vi "read_data.vi"(8 "error in (no error)":errorcluster, 11 "FeatureAgglomeration in":refnum<class "FeatureAgglomeration.lvclass">) -> (0 "error out":errorcluster, 2 "data":T1, 3 "FeatureAgglomeration out":refnum<class "FeatureAgglomeration.lvclass">)   [LabVIEW 2020, in "FeatureAgglomeration.lvclass"]
uses:
  FeatureAgglomeration.lvclass
  Controls/feature_agglomeration_data.ctl
  FeatureAgglomeration.lvclass/FeatureAgglomeration.ctl
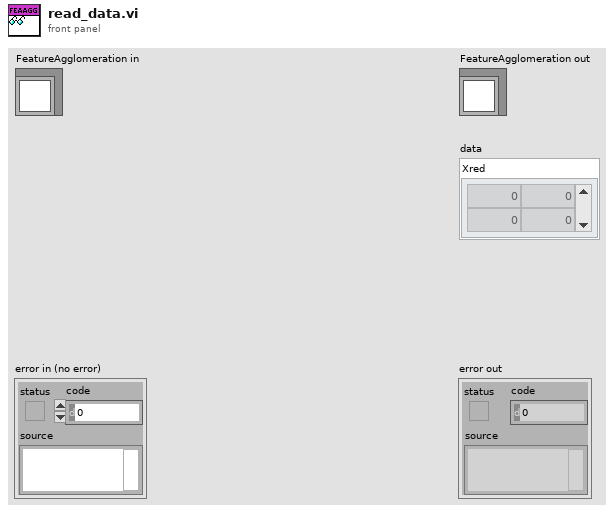
[diagram p1: front panel]
types:
  T1 = typedef "feature_agglomeration_data.ctl" = cluster{"Xred":dbl[][]}
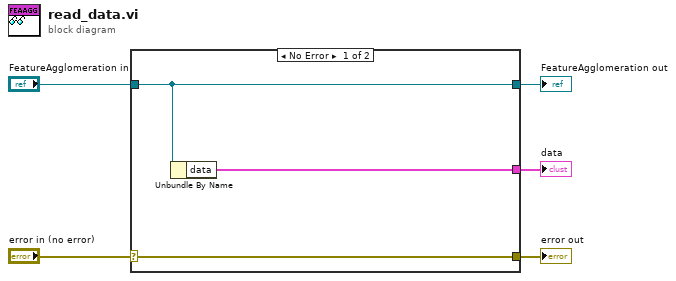
[diagram p0: block diagram]
diagram:
  n1 = case shown="No Error" "error in (no error)" {
    selector: "error in (no error)" -> [w8 w9]
    tunnel: [w8 w9] -> w4
    tunnel: [w7 w10] -> w2
    tunnel: "FeatureAgglomeration in" -> [w7 w10]
    tunnel: [w6 _] -> w1
    frame No Error {
      n2 = Unbundle By Name(w7) -> ("data"=w6:T1)
    }
    frame Error {
    }
  }
  "error out" <- w4
  "FeatureAgglomeration out" <- w2
  "data" <- w1
